vi "RSZVB Set Harmonic Relative State.vi"(8 "error in (no error)":errorcluster {"code" format="%.0x"}, 9 "Relative Harmonic Measurement (F: Off)":bool, 10 "Channel (1)":i32=1, 11 "VISA session":refnum<visa-resource-name>) -> (0 "error out":errorcluster {"code" format="%.0x"}, 3 "dup VISA session":refnum<visa-resource-name>)   [LabVIEW 2011]
doc: "This VI enables or disables the relative harmonic measurement where the harmonic is divided by the fundamental wave.\n\nRemote-control command(s):\n[SENSe<Ch>:]FREQuency:CONVersion:HARMonic:RELative ON | OFF"
panel:
  # "On\nOff"
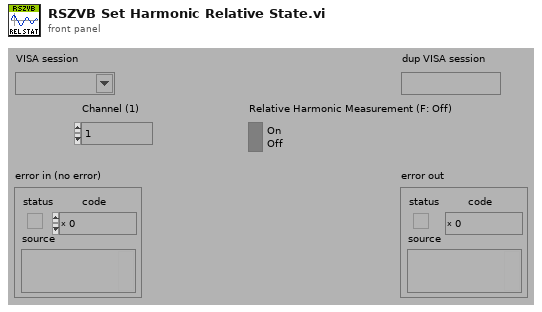
[diagram p1: front panel]
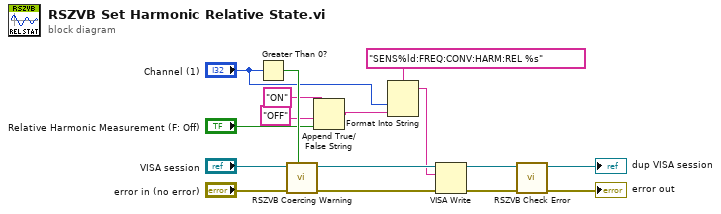
[diagram p0: block diagram]
diagram:
  n1 = Greater Than 0?(x="Channel (1)") -> (x > 0?=w10:bool)
  n2 = call "RSZVB Coercing Warning.vi"("In Range?"=w10, "error in (no error)"="error in (no error)", "VISA session"="VISA session") -> ("error out"=w14:errorcluster, "dup VISA session"=w15:refnum<visa-resource-name>)  [unwired: 7 in]
  n3 = Append True/False String(1:"Relative Harmonic Measurement (F: Off)", 2:"OFF", 3:"ON") -> (0:w7:string)  [unwired: 1 in]
  n4 = Format Into String(format string="SENS%ld:FREQ:CONV:HARM:REL %s", "Channel (1)", w7) -> (resulting string=w11:string)  [unwired: 2 in, 1 out]
  n5 = VISA Write(VISA resource name=w15, write buffer=w11, error in (no error)=w14) -> (VISA resource name out=w12:refnum<visa-resource-name>, error out=w13:errorcluster)  [unwired: 1 out]
  n6 = call "RSZVB Check Error.vi"("error in (no error)"=w13, "VISA session"=w12) -> ("error out"=→"error out":errorcluster, "dup VISA session"=→"dup VISA session":refnum<visa-resource-name>)  [unwired: 8 in]
